vi "write_pulse.vi"(8 "error in (no error)":errorcluster, 9 "type":u64, 10 "Array tdms":refnum<k34>[](array[refnum]), 11 "Array fpga":refnum<k20>[](array[refnum])) -> (0 "error in (no error) 2":errorcluster, 1 "num of pulse sent to fpga":i32, 2 "done write file":bool[](array[boolean]), 3 "tdms":refnum<k34>[](array[refnum]))   [LabVIEW 2022 SP3]
uses:
  <vilib>/Utility/error.llb/Error Cluster From Error Code.vi
  <vilib>/rvi/errors/niLvFpgaAdjustHostInterfaceError.vi
  <vilib>/rvi/interface/nirviMethod/nirviMethod.xnode
  <vilib>/FPGAPlugInAG/Dynamic/niLvFpga_WriteFifo_Dynamic.vi
  <vilib>/rvi/errors/niLvFpgaMergeErrorWithErrorCode.vi
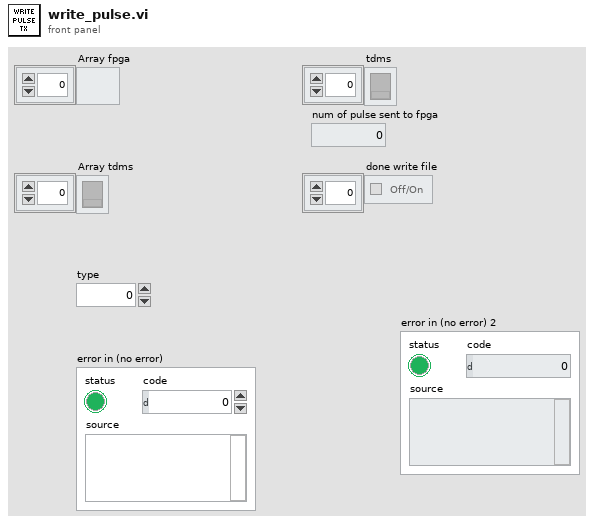
[diagram p1: front panel]
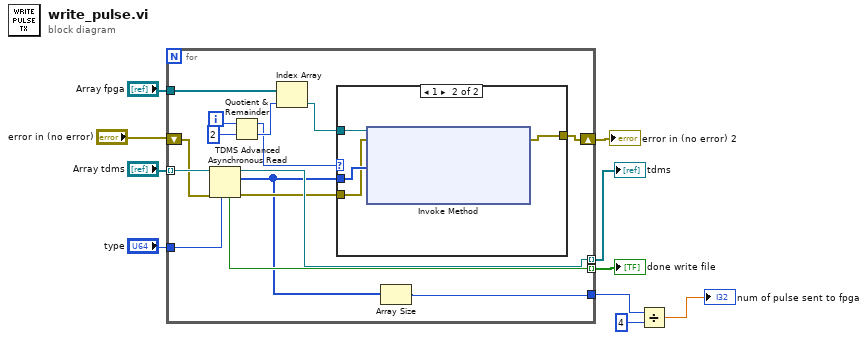
[diagram p0: block diagram]
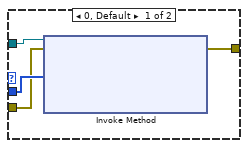
[diagram p2: hidden frame]
diagram:
  n1 = for {
    tunnel: "Array tdms" -> [w25] mode=indexing
    tunnel: "Array fpga" -> [w24]
    tunnel: "type" -> [w18]
    tunnel: [w17] -> w9 mode=indexing
    tunnel: [w16] -> w10 mode=indexing
    shift-right: [w14] -> w4
    shift-left: "error in (no error)" -> [w13]
    tunnel: [w11] -> w3
    i -> [w23]
    n2 = TDMS Advanced Asynchronous Read(6:w18, 8:w13, 11:w25) -> (0:w15:errorcluster, 2:w12:u64[], 3:w16:refnum<k34>, 4:w17:bool)
    n3 = Quotient & Remainder(x=w23, y=2) -> (x-y*floor(x/y)=w20:i32, floor(x/y)=w21:i32)
    n4 = Index Array(array=w24, index=w21) -> (element=w19:refnum<k20>)
    n5 = case shown="1" w20 {
      tunnel: w19 -> [w29 w33]
      tunnel: w12 -> [w28 w32]
      tunnel: w15 -> [w27 w31]
      tunnel: [w26 w30] -> w14
      frame 0, Default {
        n6 = xnode "Invoke Method"("FPGA VI Reference In"=w29, "error in"=w27, "Data"=w28) -> ("error out"=w26:errorcluster)  [unwired: 1 in, 2 out]
      }
      frame 1 {
        n7 = xnode "Invoke Method"("FPGA VI Reference In"=w33, "error in"=w31, "Data"=w32) -> ("error out"=w30:errorcluster)  [unwired: 1 in, 2 out]
      }
    }
    n8 = Array Size(array=w12) -> (size(s)=w11:i32)
  }
  "tdms" <- w10
  "done write file" <- w9
  "error in (no error) 2" <- w4
  n9 = Divide(x=w3, y=4) -> (x/y=→"num of pulse sent to fpga":dbl)
